vi "Set Time Data.vi"(8 "error in (no error)":errorcluster, 10 "Time Series Data":T2 {"Data Channels" format="%.2f"}, 11 "Reference in":T1) -> (0 "error out":errorcluster, 3 "Reference out":T1)   [LabVIEW 2013, in "Impulse Data.lvclass"]
uses:
  Impulse Data.lvclass
  Instance handle.ctl
  Impulse Data.lvclass/Impulse Data.ctl
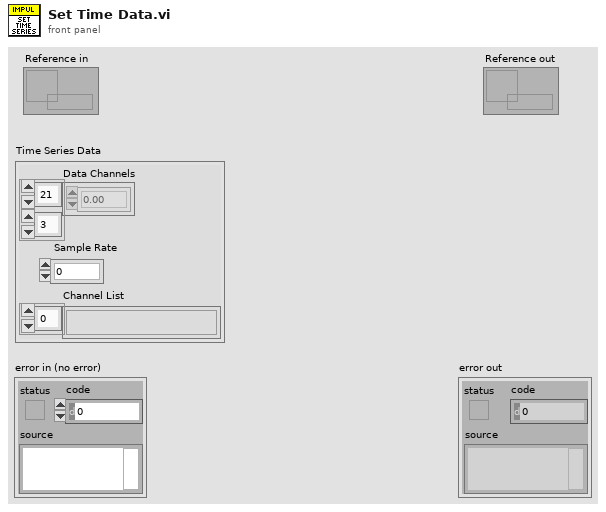
[diagram p1: front panel]
types:
  T1 = typedef "Impulse Data.lvclass/Instance handle.ctl" = refnum<data-value>
  T2 = cluster{"Data Channels":dbl[][], "Sample Rate":i32, "Channel List":string[]}
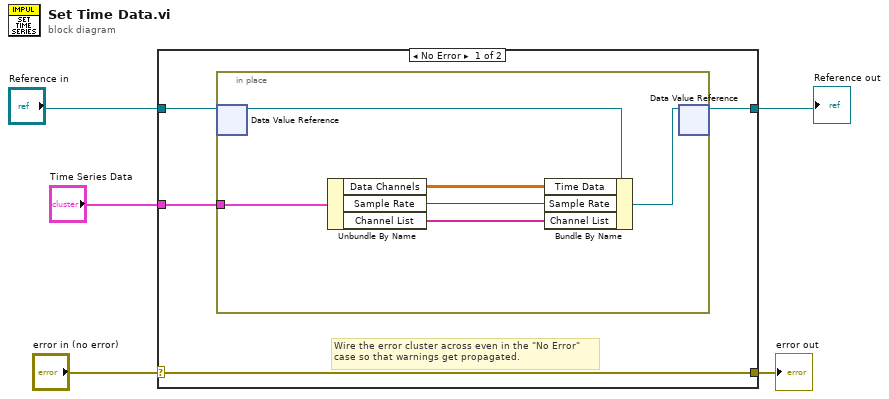
[diagram p0: block diagram]
diagram:
  n1 = case shown="No Error" "error in (no error)" {
    selector: "error in (no error)" -> [w9 w17]
    tunnel: [w9 w17] -> w4
    tunnel: [w6 w16] -> w1
    tunnel: "Reference in" -> [w7 w16]
    tunnel: "Time Series Data" -> [w8 _]
    frame No Error {
      # "Wire the error cluster across even in the \"No Error\"\ncase so that warnings get propagated."
      n2 = in-place {
        in-place-border: w8 -> [w15]
        n3 = in-place-dvr #1(w7) -> (w10:refnum<class "Impulse Data.lvclass">)  [unwired: 1 out]
        n4 = Unbundle By Name(w15) -> ("Data Channels"=w12:dbl[][], "Sample Rate"=w14:i32, "Channel List"=w13:string[])
        n5 = Bundle By Name(cluster=w10, "Time Data"=w12, "Sample Rate"=w14, "Channel List"=w13) -> (w11:refnum<class "Impulse Data.lvclass">)
        n6 = in-place-dvr #1(w11) -> (w6:T1)  [unwired: 1 out]
      }
    }
    frame Error {
    }
  }
  "error out" <- w4
  "Reference out" <- w1
